vi "IdentifyBlobPoly.vi"   [LabVIEW 2024]
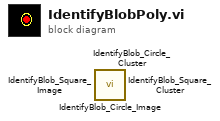
[diagram p0: block diagram]
diagram:
  n1 = call <userlib>:"IdentifyBlob_Circle_Image.vi"() -> ()  [unwired: 4 in, 1 out]
  n2 = call <userlib>:"IdentifyBlob_Circle_Cluster.vi"() -> ()  [unwired: 4 in, 1 out]
  n3 = call <userlib>:"IdentifyBlob_Square_Image.vi"() -> ()  [unwired: 4 in, 1 out]
  n4 = call <userlib>:"IdentifyBlob_Square_Cluster.vi"() -> ()  [unwired: 4 in, 1 out]
